vi "Init.vi"() -> (0 "Error Out":errorcluster, 1 "FPGA VI Reference Out":refnum<k20>)   [LabVIEW 2018]
doc: "Initialize all values"
uses:
  Type Defs/State Machine.ctl
  Type Defs/Global Action.ctl
  <vilib>/FPGAPlugInAG/sbRIO-9607/niLvFpga_Open_sbRIO-9607.vi
  <vilib>/rvi/interface/common/dynamic/niFpgaDynamicAddResources.vi
  <vilib>/rvi/interface/nirviOpenFPGA/nirviOpenFPGA.xnode
  FPGA Bitfiles/NewDAS_FPGATarget_FPGAMain_Tp2qXx1cKwU.lvbitx
  FPGA/FPGA Main.vi
panel:
  out "FilePath":path
  out "FPGA Version":dbl
  in  "Force Simulation":bool
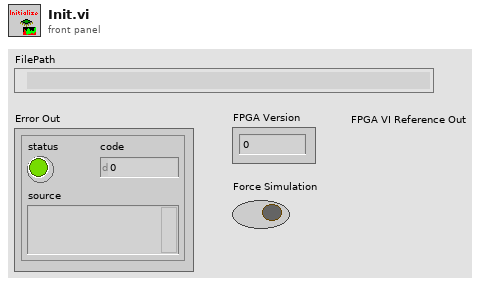
[diagram p1: front panel]
types:
  T1 = typedef "State Machine.ctl" = enum16{"Case 0", "Case 1", "Case 2", "Case 3", "Case 4", "Case 5", "Case 6", "Case 7", "Case 8", "Case 9", "Case 10", "Case 11", "Case 12", "Case 13", "Case 14", "Case 15", "Case 16", "Error", "Exit"}
  T2 = typedef "Global Action.ctl" = enum16{"Write", "Read"}
  T3 = typedef "RT Parameters.ctl" = cluster{"Configuration":T4, "Startup Options":cluster{"Door":bool, "Curtain":bool, "Pressure":bool, "Turbo":bool, "SysPoll":bool, "GasFlag":bool, "SourceExhaust":bool}, "ADC Table":T6[], "Q2 POL":bool, "Q1 POL":bool, "Simulation":bool, "Exhsuast Gas Error":bool, "Electronics ON":bool, "Single Source":bool, "L pump ON":bool, "Laybold":bool, "Ignore Error":bool, "Scan Param":bool, "Tuning Error":bool, "RT Time":dbl, "Error Msg":string, "Connected?":bool, "Ready":bool, "Fault":bool}
  T4 = typedef "Main Configration.ctl" = cluster{"Table":T5[], "Instrument":string[]}
  T5 = typedef "Configration.ctl" = cluster{"Name":string, "Ch#":u8, "Min":dbl, "Max":dbl, "Def+":dbl, "Def-":dbl, "Offset":dbl, "Slope":dbl, "Type":u8, "Description":string, "SettleT":dbl}
  T6 = typedef "RT Configuration.ctl" = cluster{"Name":string, "Ch#":u8, "Min":dbl, "Max":dbl, "Def+":dbl, "Def-":dbl, "Offset":dbl, "Slope":dbl, "Type":u8, "Description":string, "SettleT":dbl}
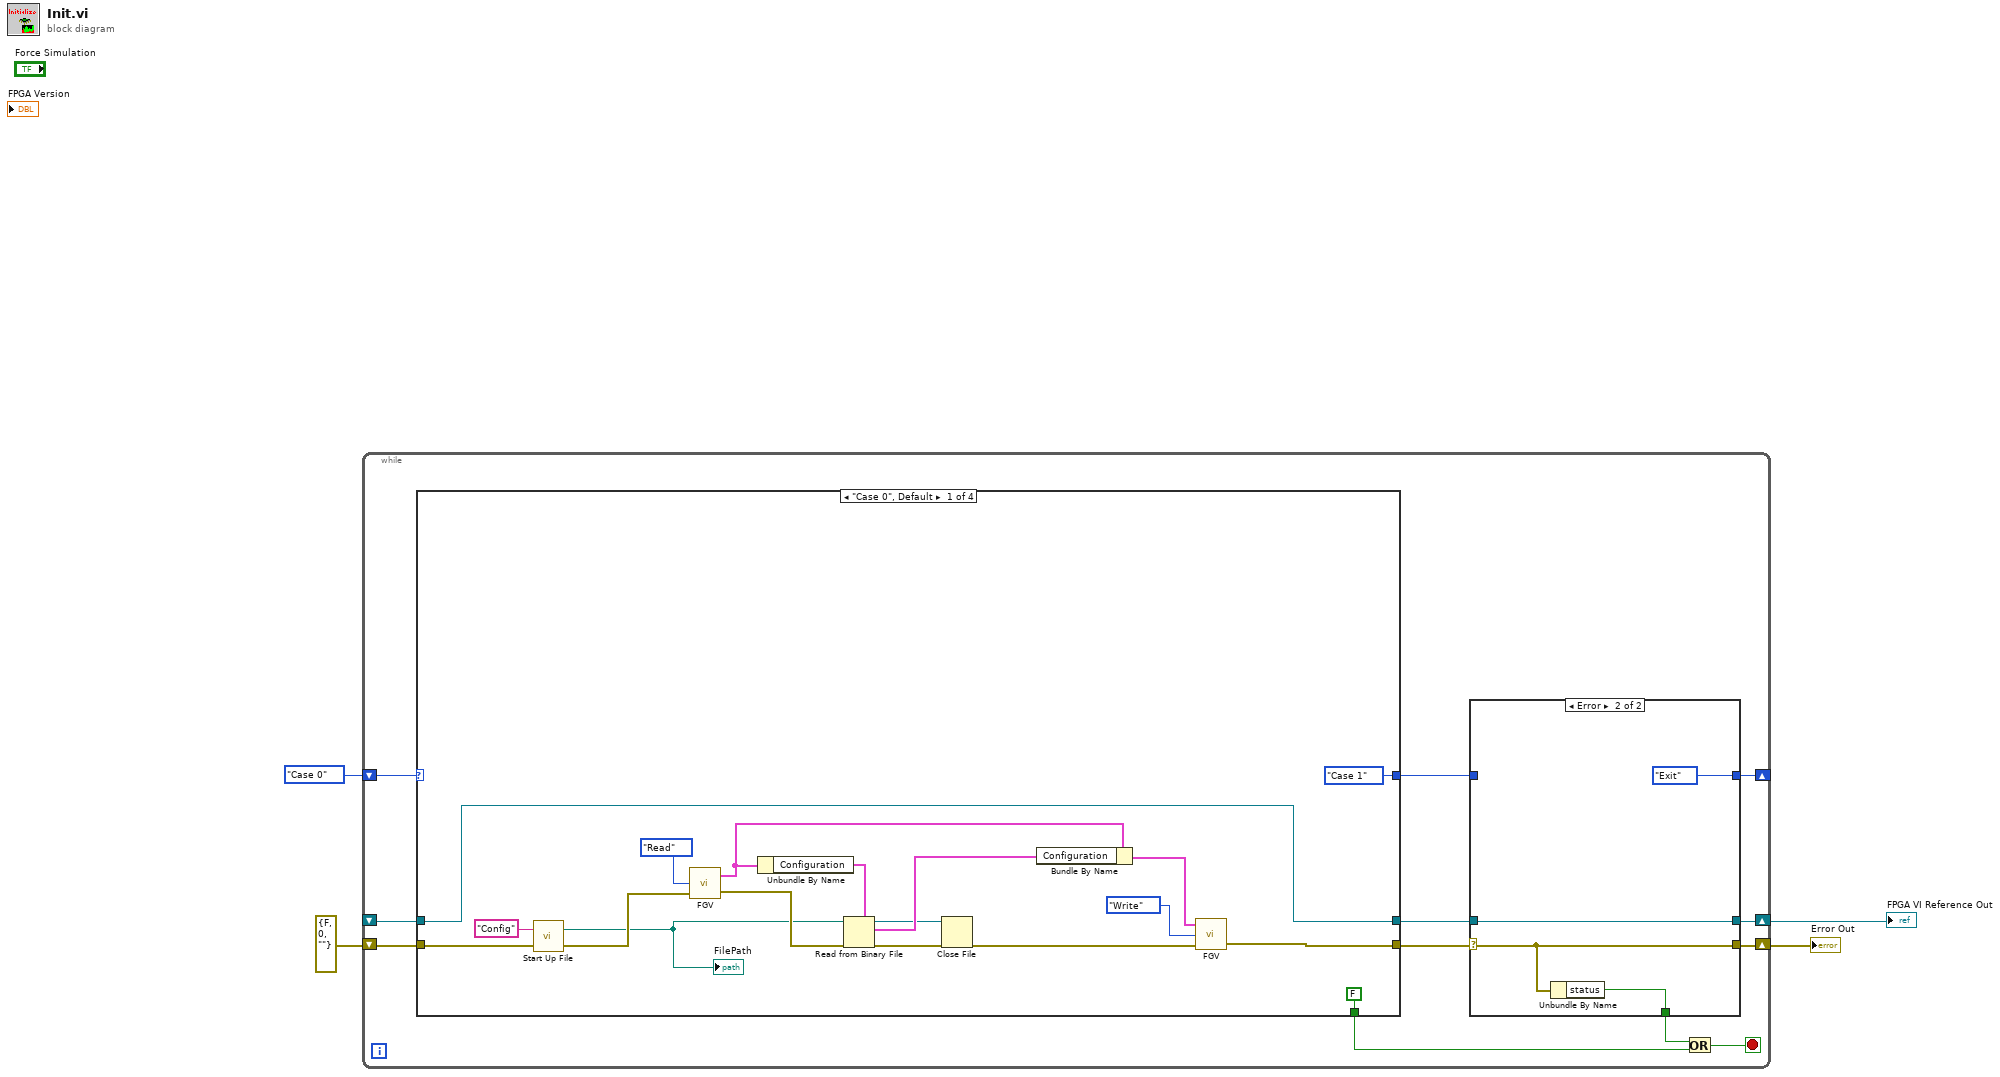
[diagram p0: block diagram]
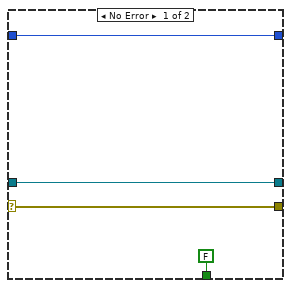
[diagram p2: hidden frame]
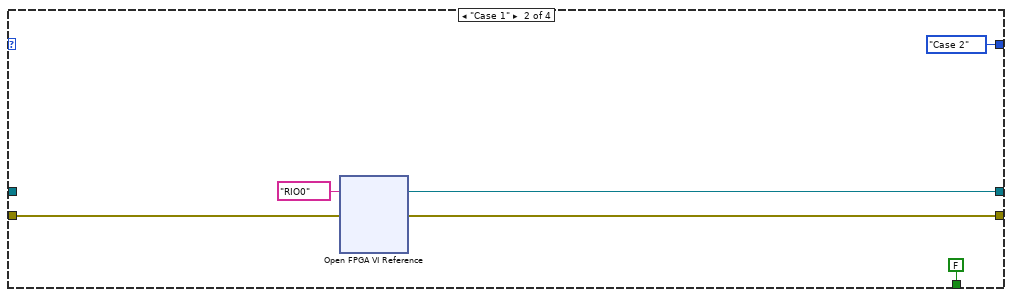
[diagram p3: hidden frame]
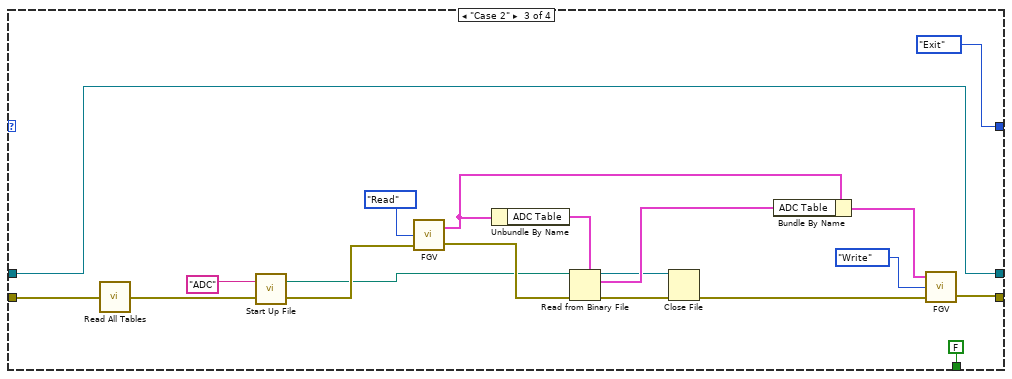
[diagram p4: hidden frame]
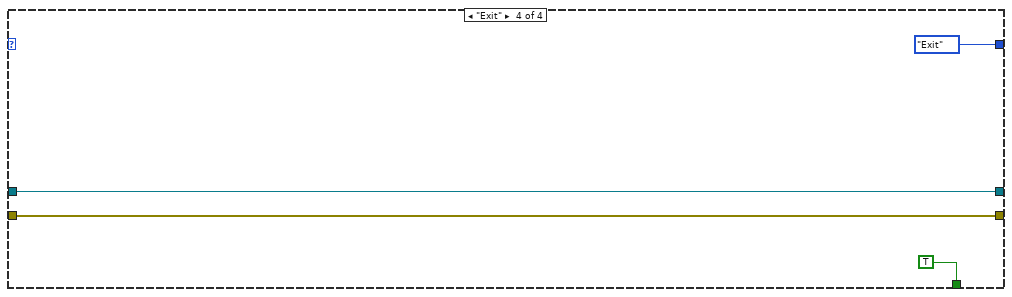
[diagram p5: hidden frame]
diagram:
  n1 = while {
    shift-right: [w15] -> _
    shift-left: State_Machine."Case 0" ("Enum") -> [w16]
    shift-right: [w13] -> w3
    shift-left: errorcluster {"status"=FALSE, "code"=0, "source"=""} ("error IO") -> [w12]
    shift-right: [w6] -> w1
    shift-left: _ -> [w5]
    stop <- w10 stop-if-true
    n2 = case shown="\"Case 0\", Default" w16 {
      tunnel: [w33 w45 w51 w70] -> w14
      tunnel: w12 -> [w37 w46 w67 w70]
      tunnel: [FALSE FALSE FALSE TRUE] -> w9
      tunnel: [State_Machine."Case 1" ("Enum") State_Machine."Case 2" ("Enum") State_Machine."Exit" ("Enum") State_Machine."Exit" ("Enum")] -> w8
      tunnel: [w25 w44 w49 w68] -> w7
      tunnel: w5 -> [w25 _ w49 w68]
      frame "Case 0", Default {
        n3 = call "Start Up File.vi"("error in (no error)"=w37, "FileName"="Config" ("key")) -> ("error out"=w40:errorcluster, "FilePath"=w38:path)
        "FilePath" <- w38
        n4 = call "FGV.vi"("Error In"=w40, "Action"=Global_Action."Read") -> ("Error Out"=w39:errorcluster, "Parameters Out"=w31:T3)  [unwired: 1 in]
        n5 = Unbundle By Name(w31) -> ("Configuration"=w32:T4)
        n6 = Read from Binary File(5:w32, 8:w39, 11:w38) -> (0:w26:errorcluster, 2:w29:T4, 3:w27:refnum<file>)  [unwired: 4 out]
        n7 = Close File(refnum=w27, error in=w26) -> (error out=w34:errorcluster)  [unwired: 1 out]
        n8 = Bundle By Name(cluster=w31, "Configuration"=w29) -> (w30:T3)
        n9 = call "FGV.vi"("Error In"=w34, "Action"=Global_Action."Write", "Parameters In"=w30) -> ("Error Out"=w33:errorcluster)  [unwired: 1 out]
      }
      frame "Case 1" {
        n10 = xnode "Open FPGA VI Reference"("error in"=w46, "resource name"=tag "RIO0") -> ("FPGA VI Reference Out"=w44:refnum<k20>, "error out"=w45:errorcluster)
      }
      frame "Case 2" {
        n11 = call "Read All Tables.vi"("Error In"=w67) -> ("Error Out"=w52:errorcluster)
        n12 = call "Start Up File.vi"("error in (no error)"=w52, "FileName"="ADC" ("key")) -> ("error out"=w63:errorcluster, "FilePath"=w61:path)
        n13 = call "FGV.vi"("Error In"=w63, "Action"=Global_Action."Read") -> ("Error Out"=w62:errorcluster, "Parameters Out"=w58:T3)  [unwired: 1 in]
        n14 = Unbundle By Name(w58) -> ("ADC Table"=w59:T6[])
        n15 = Read from Binary File(5:w59, 8:w62, 11:w61) -> (0:w53:errorcluster, 2:w56:T6[], 3:w54:refnum<file>)  [unwired: 4 out]
        n16 = Close File(refnum=w54, error in=w53) -> (error out=w60:errorcluster)  [unwired: 1 out]
        n17 = Bundle By Name(cluster=w58, "ADC Table"=w56) -> (w57:T3)
        n18 = call "FGV.vi"("Error In"=w60, "Action"=Global_Action."Write", "Parameters In"=w57) -> ("Error Out"=w51:errorcluster)  [unwired: 1 out]
      }
      frame "Exit" {
      }
    }
    n19 = case shown="Error" w14 {
      selector: w14 -> [w20 w23]
      tunnel: [w18 State_Machine."Exit" ("Enum")] -> w15
      tunnel: [w20 w23] -> w13
      tunnel: [FALSE ("status") w22] -> w11
      tunnel: w8 -> [w18 _]
      tunnel: w7 -> [w17 w21]
      tunnel: [w17 w21] -> w6
      frame No Error {
      }
      frame Error {
        n20 = Unbundle By Name(w23) -> ("status"=w22:bool)
      }
    }
    n21 = Or(x=w11, y=w9) -> (x .or. y?=w10:bool)
  }
  "Error Out" <- w3
  "FPGA VI Reference Out" <- w1
